vi "DeltaE(2000).vi"(1 "L*a*b Colors":T1) -> (0 "Delta E":dbl)   [LabVIEW 2013]
panel:
  out "D L'":dbl
  out "D C'":dbl
  out "Rt":dbl
  out "Sc":dbl
  out "Sh":dbl
  out "Sl":dbl
  out "DH":dbl
  out "H'":dbl
  out "T":dbl
  out "D h'":dbl
  out "L'_":dbl
  out "C'_":dbl
  out "C2'":dbl
  out "C1'":dbl
  out "a2'":dbl
  out "a1'":dbl
  out "G":dbl
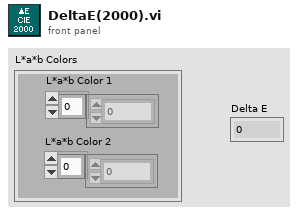
[diagram p1: front panel]
types:
  T1 = cluster{"L*a*b Color 1":dbl[], "L*a*b Color 2":dbl[]}
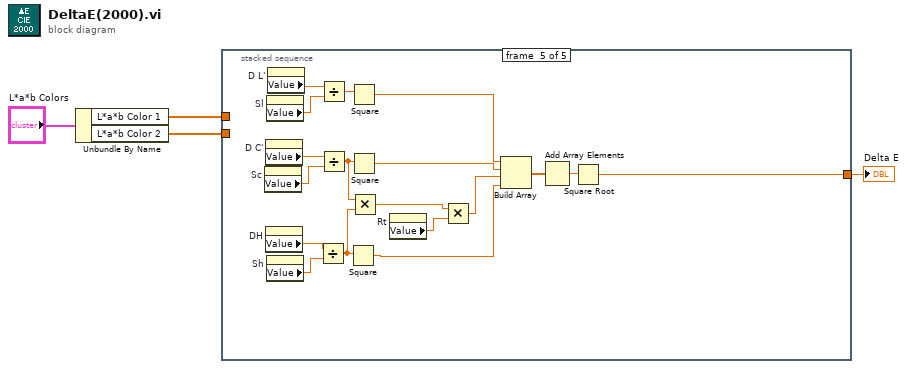
[diagram p0: block diagram]
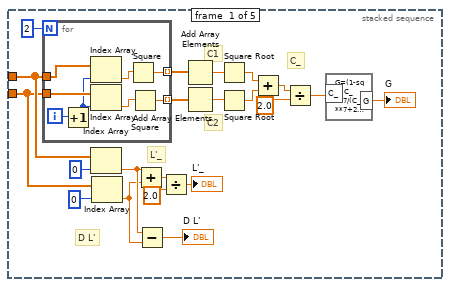
[diagram p2: hidden frame]
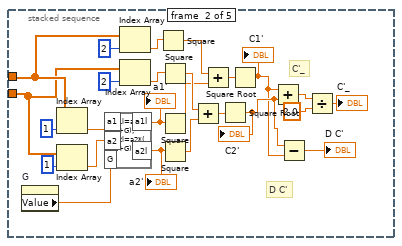
[diagram p3: hidden frame]
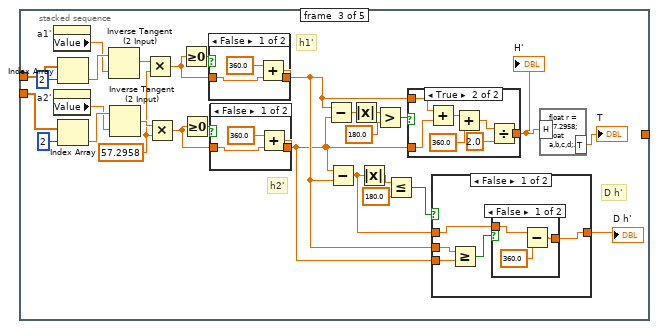
[diagram p4: hidden frame]
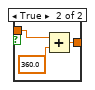
[diagram p5: hidden frame]
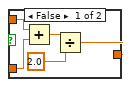
[diagram p7: hidden frame]
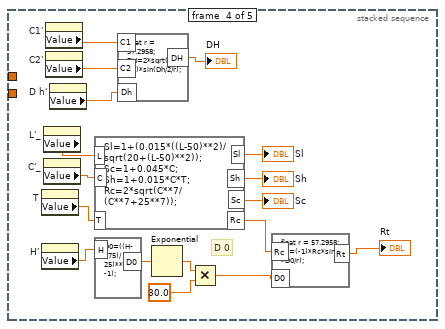
[diagram p10: hidden frame]
diagram:
  n1 = Unbundle By Name("L*a*b Colors") -> ("L*a*b Color 1"=w3:dbl[], "L*a*b Color 2"=w2:dbl[])
  n2 = stacked-sequence {
    tunnel: w3 -> [w16 w51 w86 _ _]
    tunnel: w2 -> [w15 w50 w83 _ _]
    tunnel: [_ _ _ _ w136] -> w1
    frame #0 {
      # "D L'"
      # "L'_"
      # "C_"
      # "C2"
      # "C1"
      n3 = for {
        N: 2 -> [_]
        tunnel: w16 -> [w32]
        tunnel: w15 -> [w31]
        tunnel: [w27] -> w24 mode=indexing
        tunnel: [w26] -> w23 mode=indexing
        i -> [w33]
        n4 = Increment(x=w33) -> (x+1=w30:i32)
        n5 = Index Array(array=w32, index=w30) -> (element=w29:dbl)
        n6 = Index Array(array=w31, index=w30) -> (element=w28:dbl)
        n7 = Square(x=w29) -> (x^2=w27:dbl)
        n8 = Square(x=w28) -> (x^2=w26:dbl)
      }
      n9 = Index Array(array=w16, index=0) -> (element=w10:dbl)
      n10 = Index Array(array=w15, index=0) -> (element=w9:dbl)
      n11 = Add(x=w10, y=w9) -> (x+y=w12:dbl)
      n12 = Subtract(x=w10, y=w9) -> (x-y=→"D L'":dbl)
      n13 = Divide(x=w12, y=2.0) -> (x/y=→"L'_":dbl)
      n14 = Add Array Elements(numeric array=w24) -> (sum=w22:dbl)
      n15 = Add Array Elements(numeric array=w23) -> (sum=w21:dbl)
      n16 = Square Root(x=w22) -> (sqrt(x)=w20:dbl)
      n17 = Square Root(x=w21) -> (sqrt(x)=w19:dbl)
      n18 = Add(x=w20, y=w19) -> (x+y=w18:dbl)
      n19 = Divide(x=w18, y=2.0) -> (x/y=w8:dbl)
      n20 = formula code="G=(1-sqrt(C_**7/(C_**7+25**7)))/2;"("C_"=w8) -> ("G"=→"G":dbl)
    }
    frame #1 {
      # "D C'"
      # "C'_"
      n21 = property on="G" class="DigNum (strict)"() -> ("Value"=w54:dbl)  [unwired: 2 in, 2 out]
      n22 = Index Array(array=w51, index=1) -> (element=w56:dbl)
      n23 = Index Array(array=w50, index=1) -> (element=w55:dbl)
      n24 = formula code="a1l=a1*(1+G);\na2l=a2*(1+G);"("a1"=w56, "a2"=w55, "G"=w54) -> ("a1l"=w52:dbl, "a2l"=w53:dbl)
      "a1'" <- w52
      "a2'" <- w53
      n25 = Index Array(array=w51, index=2) -> (element=w47:dbl)
      n26 = Index Array(array=w50, index=2) -> (element=w46:dbl)
      n27 = Square(x=w47) -> (x^2=w43:dbl)
      n28 = Square(x=w46) -> (x^2=w45:dbl)
      n29 = Square(x=w52) -> (x^2=w42:dbl)
      n30 = Square(x=w53) -> (x^2=w44:dbl)
      n31 = Add(x=w45, y=w44) -> (x+y=w41:dbl)
      n32 = Add(x=w43, y=w42) -> (x+y=w40:dbl)
      n33 = Square Root(x=w41) -> (sqrt(x)=w37:dbl)
      "C2'" <- w37
      n34 = Square Root(x=w40) -> (sqrt(x)=w36:dbl)
      "C1'" <- w36
      n35 = Add(x=w36, y=w37) -> (x+y=w39:dbl)
      n36 = Subtract(x=w37, y=w36) -> (x-y=→"D C'":dbl)
      n37 = Divide(x=w39, y=2.0) -> (x/y=→"C'_":dbl)
    }
    frame #2 {
      w62 = 57.2958
      # "D h'"
      # "h2'"
      # "h1'"
      n38 = property on="a1'" class="DigNum (strict)"() -> ("Value"=w64:dbl)  [unwired: 2 in, 2 out]
      n39 = property on="a2'" class="DigNum (strict)"() -> ("Value"=w68:dbl)  [unwired: 2 in, 2 out]
      n40 = Index Array(array=w86, index=2) -> (element=w65:dbl)
      n41 = Index Array(array=w83, index=2) -> (element=w69:dbl)
      n42 = Inverse Tangent (2 Input)(1:w64, 2:w65) -> (0:w63:dbl)
      n43 = Inverse Tangent (2 Input)(1:w68, 2:w69) -> (0:w67:dbl)
      n44 = Multiply(x=w63, y=w62) -> (x*y=w61:dbl)
      n45 = Multiply(x=w67, y=w62) -> (x*y=w66:dbl)
      n46 = Greater Or Equal To 0?(x=w61) -> (x >= 0?=w82:bool)
      n47 = Greater Or Equal To 0?(x=w66) -> (x >= 0?=w81:bool)
      n48 = case shown="False" w82 {
        tunnel: w61 -> [w116 w118]
        tunnel: [w115 w118] -> w72
        frame False {
          n49 = Add(x=360.0, y=w116) -> (x+y=w115:dbl)
        }
        frame True {
        }
      }
      n50 = case shown="False" w81 {
        tunnel: w66 -> [w112 w114]
        tunnel: [w111 w114] -> w71
        frame False {
          n51 = Add(x=360.0, y=w112) -> (x+y=w111:dbl)
        }
        frame True {
        }
      }
      n52 = Subtract(x=w72, y=w71) -> (x-y=w80:dbl)
      n53 = Subtract(x=w71, y=w72) -> (x-y=w73:dbl)
      n54 = Absolute Value(x=w80) -> (abs(x)=w79:dbl)
      n55 = Absolute Value(x=w73) -> (abs(x)=w76:dbl)
      n56 = Greater?(x=w79, y=180.0) -> (0:w77:bool)
      n57 = Less Or Equal?(x=w76, y=180.0) -> (x <= y?=w74:bool)
      n58 = case shown="True" w77 {
        tunnel: w72 -> [w103 w110]
        tunnel: w71 -> [w102 w109]
        tunnel: [w99 w104] -> w59
        frame False {
          n59 = Add(x=w103, y=w102) -> (x+y=w101:dbl)
          n60 = Divide(x=w101, y=2.0) -> (x/y=w99:dbl)
        }
        frame True {
          n61 = Add(x=w110, y=w109) -> (x+y=w108:dbl)
          n62 = Add(x=w108, y=360.0) -> (x+y=w106:dbl)
          n63 = Divide(x=w106, y=2.0) -> (x/y=w104:dbl)
        }
      }
      "H'" <- w59
      n64 = case shown="False" w74 {
        tunnel: w73 -> [w88 w98]
        tunnel: [w87 w98] -> w70
        tunnel: w72 -> [w90 _]
        tunnel: w71 -> [w91 _]
        frame False {
          n65 = Greater Or Equal?(x=w90, y=w91) -> (x >= y?=w89:bool)
          n66 = case shown="False" w89 {
            tunnel: w88 -> [w94 w97]
            tunnel: [w92 w96] -> w87
            frame False {
              n67 = Subtract(x=w94, y=360.0) -> (x-y=w92:dbl)
            }
            frame True {
              n68 = Add(x=w97, y=360.0) -> (x+y=w96:dbl)
            }
          }
        }
        frame True {
        }
      }
      "D h'" <- w70
      n69 = formula code="float r = 57.2958;\nfloat a,b,c,d;\na = 0.17*cos((H-30)/r);\nb = 0.24*cos(2*H/r);\nc = 0.32*cos((3*H+6)/r);\nd = 0.2*cos((4*H-63)/r);\nT=1-a+b+c-d;"("H"=w59) -> ("T"=→"T":dbl)
    }
    frame #3 {
      # "D 0"
      n70 = property on="T" class="DigNum (strict)"() -> ("Value"=w133:dbl)  [unwired: 2 in, 2 out]
      n71 = property on="H'" class="DigNum (strict)"() -> ("Value"=w132:dbl)  [unwired: 2 in, 2 out]
      n72 = property on="L'_" class="DigNum (strict)"() -> ("Value"=w135:dbl)  [unwired: 2 in, 2 out]
      n73 = property on="C'_" class="DigNum (strict)"() -> ("Value"=w134:dbl)  [unwired: 2 in, 2 out]
      n74 = property on="C1'" class="DigNum (strict)"() -> ("Value"=w124:dbl)  [unwired: 2 in, 2 out]
      n75 = property on="C2'" class="DigNum (strict)"() -> ("Value"=w123:dbl)  [unwired: 2 in, 2 out]
      n76 = property on="D h'" class="DigNum (strict)"() -> ("Value"=w122:dbl)  [unwired: 2 in, 2 out]
      n77 = formula code="Sl=1+(0.015*((L-50)**2)/sqrt(20+(L-50)**2));\nSc=1+0.045*C;\nSh=1+0.015*C*T;\nRc=2*sqrt(C**7/(C**7+25**7));"("L"=w135, "C"=w134, "T"=w133) -> ("Sl"=→"Sl":dbl, "Sh"=→"Sh":dbl, "Sc"=→"Sc":dbl, "Rc"=w121:dbl)
      n78 = formula code="D0=((H-275)/25)**2*(-1);"("H"=w132) -> ("D0"=w131:dbl)
      n79 = formula code="float r = 57.2958;\nDH=2*sqrt(C1*C2)*sin(Dh/2/r);"("C1"=w124, "C2"=w123, "Dh"=w122) -> ("DH"=→"DH":dbl)
      n80 = Exponential(1:w131) -> (0:w130:dbl)
      n81 = Multiply(x=w130, y=30.0) -> (x*y=w120:dbl)
      n82 = formula code="float r = 57.2958;\nRt=(-1)*Rc*sin(2*D0/r);"("Rc"=w121, "D0"=w120) -> ("Rt"=→"Rt":dbl)
    }
    frame #4 {
      n83 = property on="Sc" class="DigNum (strict)"() -> ("Value"=w150:dbl)  [unwired: 2 in, 2 out]
      n84 = property on="D C'" class="DigNum (strict)"() -> ("Value"=w151:dbl)  [unwired: 2 in, 2 out]
      n85 = property on="DH" class="DigNum (strict)"() -> ("Value"=w149:dbl)  [unwired: 2 in, 2 out]
      n86 = property on="Sl" class="DigNum (strict)"() -> ("Value"=w152:dbl)  [unwired: 2 in, 2 out]
      n87 = property on="Sh" class="DigNum (strict)"() -> ("Value"=w148:dbl)  [unwired: 2 in, 2 out]
      n88 = property on="D L'" class="DigNum (strict)"() -> ("Value"=w153:dbl)  [unwired: 2 in, 2 out]
      n89 = Divide(x=w149, y=w148) -> (x/y=w145:dbl)
      n90 = Divide(x=w153, y=w152) -> (x/y=w147:dbl)
      n91 = Divide(x=w151, y=w150) -> (x/y=w146:dbl)
      n92 = Square(x=w145) -> (x^2=w142:dbl)
      n93 = Square(x=w147) -> (x^2=w139:dbl)
      n94 = Square(x=w146) -> (x^2=w140:dbl)
      n95 = Multiply(x=w146, y=w145) -> (x*y=w143:dbl)
      n96 = property on="Rt" class="DigNum (strict)"() -> ("Value"=w144:dbl)  [unwired: 2 in, 2 out]
      n97 = Multiply(x=w143, y=w144) -> (x*y=w141:dbl)
      n98 = Build Array(w139, w140, w141, w142) -> (w138:dbl[])
      n99 = Add Array Elements(numeric array=w138) -> (sum=w137:dbl)
      n100 = Square Root(x=w137) -> (sqrt(x)=w136:dbl)
    }
  }
  "Delta E" <- w1
